vi "GEOM_GetTotData.vi"(10 "CorrectedFPA":T1[](array[typedef])) -> (1 "tot data rows":i32, 2 "tot data columns":i32)   [LabVIEW 2016]
uses:
  GEOM_CorrectedFPA.ctl
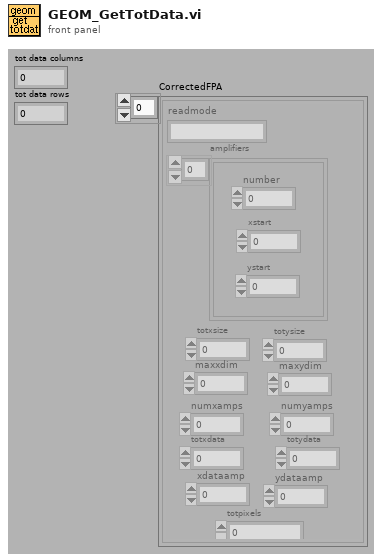
[diagram p1: front panel]
types:
  T1 = typedef "GEOM_CorrectedFPA.ctl" = cluster{"readmode":string, "amplifiers":cluster{"number":i32, "xstart":i32, "ystart":i32}[], "totxsize":i32, "totysize":i32, "maxxdim":i32, "maxydim":i32, "numxamps":i32, "numyamps":i32, "totxdata":i32, "totydata":i32, "xdataamp":i32, "ydataamp":i32, "totpixels":i32}
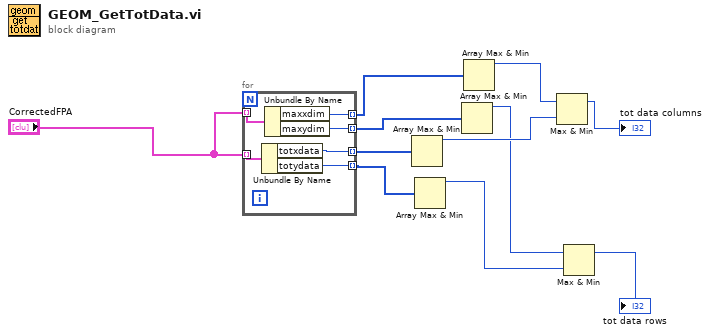
[diagram p0: block diagram]
diagram:
  n1 = for {
    tunnel: "CorrectedFPA" -> [w17] mode=indexing
    tunnel: [w16] -> w11 mode=indexing
    tunnel: [w15] -> w10 mode=indexing
    tunnel: "CorrectedFPA" -> [w14] mode=indexing
    tunnel: [w13] -> w8 mode=indexing
    tunnel: [w12] -> w7 mode=indexing
    n2 = Unbundle By Name(w17) -> ("totxdata"=w16:i32, "totydata"=w15:i32)
    n3 = Unbundle By Name(w14) -> ("maxxdim"=w13:i32, "maxydim"=w12:i32)
  }
  n4 = Array Max & Min(array=w11) -> (max value=w5:i32)  [unwired: 3 out]
  n5 = Array Max & Min(array=w10) -> (max value=w2:i32)  [unwired: 3 out]
  n6 = Array Max & Min(array=w7) -> (max value=w3:i32)  [unwired: 3 out]
  n7 = Array Max & Min(array=w8) -> (max value=w6:i32)  [unwired: 3 out]
  n8 = Max & Min(x=w6, y=w5) -> (max(x,y)=→"tot data columns":i32)  [unwired: 1 out]
  n9 = Max & Min(x=w3, y=w2) -> (max(x,y)=→"tot data rows":i32)  [unwired: 1 out]
